vi "DSF.Engine.Pool.Plugin Interface.Get Plugin Interfaces.vi"(11 "Plugin Interface Pool in":refnum<class "DSF.Engine.Pool.Plugin Interface.lvclass">) -> (2 "Plugin Interfaces":refnum<class "DSF.Engine.Interface.Plugin.lvclass">[](array[class]), 3 "Plugin Interface Pool out":refnum<class "DSF.Engine.Pool.Plugin Interface.lvclass">)   [LabVIEW 2016, in "DSF.Engine.lvlib" / "DSF.Engine.Pool.Plugin Interface.lvclass"]
uses:
  DSF.Engine.Pool.Plugin Interface.lvclass
  Interface/DSF.Engine.Interface.Plugin.lvclass
  DSF.Engine.Pool.Plugin Interface.lvclass/DSF.Engine.Pool.Plugin Interface.ctl
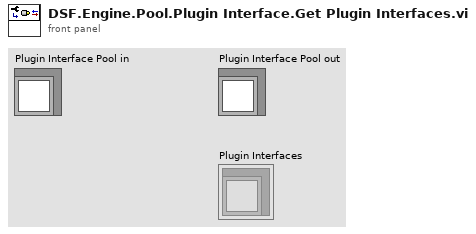
[diagram p1: front panel]
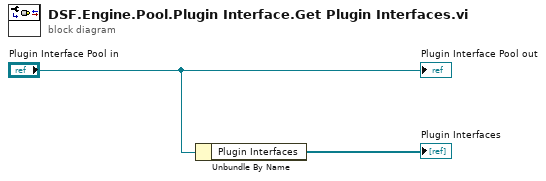
[diagram p0: block diagram]
diagram:
  n1 = Unbundle By Name("Plugin Interface Pool in") -> ("Plugin Interfaces"=→"Plugin Interfaces":refnum<class "DSF.Engine.Interface.Plugin.lvclass">[])
  "Plugin Interface Pool out" <- "Plugin Interface Pool in"
